vi "UI Config Controls.vi"(8 "Error In":errorcluster, 10 "UI Configuration":T1, 11 "UI Data":T2) -> (0 "Error Out":errorcluster, 3 "UI Data 2":T2)   [LabVIEW 2015]
uses:
  controls/UI Data.ctl
  controls/Instruments.ctl
  controls/UI Config.ctl
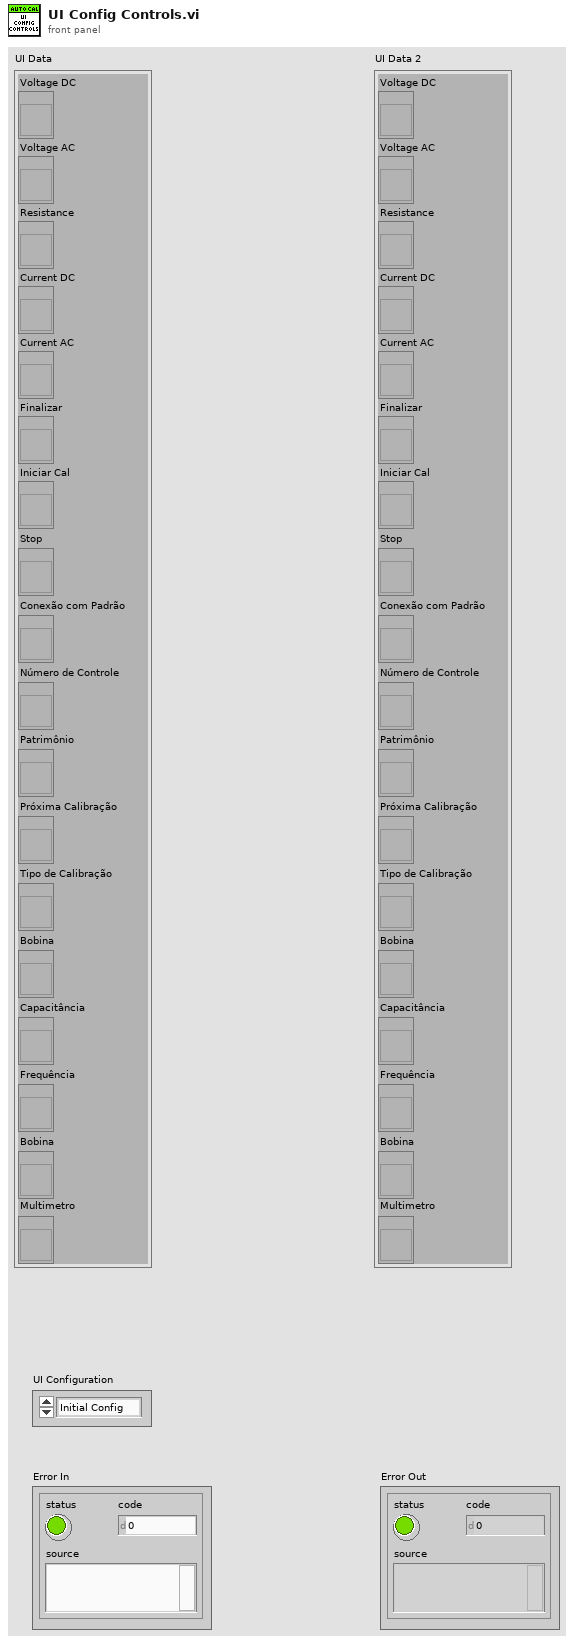
[diagram p1: front panel]
types:
  T1 = typedef "UI Config.ctl" = enum16{"Initial Config", "Calibration Config"}
  T2 = typedef "UI Data.ctl" = cluster{"Voltage DC":refnum<vi>, "Voltage AC":refnum<vi>, "Resistance":refnum<vi>, "Current DC":refnum<vi>, "Current AC":refnum<vi>, "Finalizar":refnum<vi>, "Iniciar Cal":refnum<vi>, "Stop":refnum<vi>, "Conexão com Padrão":refnum<vi>, "Número de Controle":refnum<vi>, "Patrimônio":refnum<vi>, "Próxima Calibração":refnum<vi>, "Tipo de Calibração":refnum<vi>, "Bobina":refnum<vi>, "Capacitância":refnum<vi>, "Frequência":refnum<vi>, "Bobina":refnum<vi>, "Multimetro":refnum<vi>}
  T3 = enum8{"Enabled", "Disabled", "Disabled and Grayed Out"}
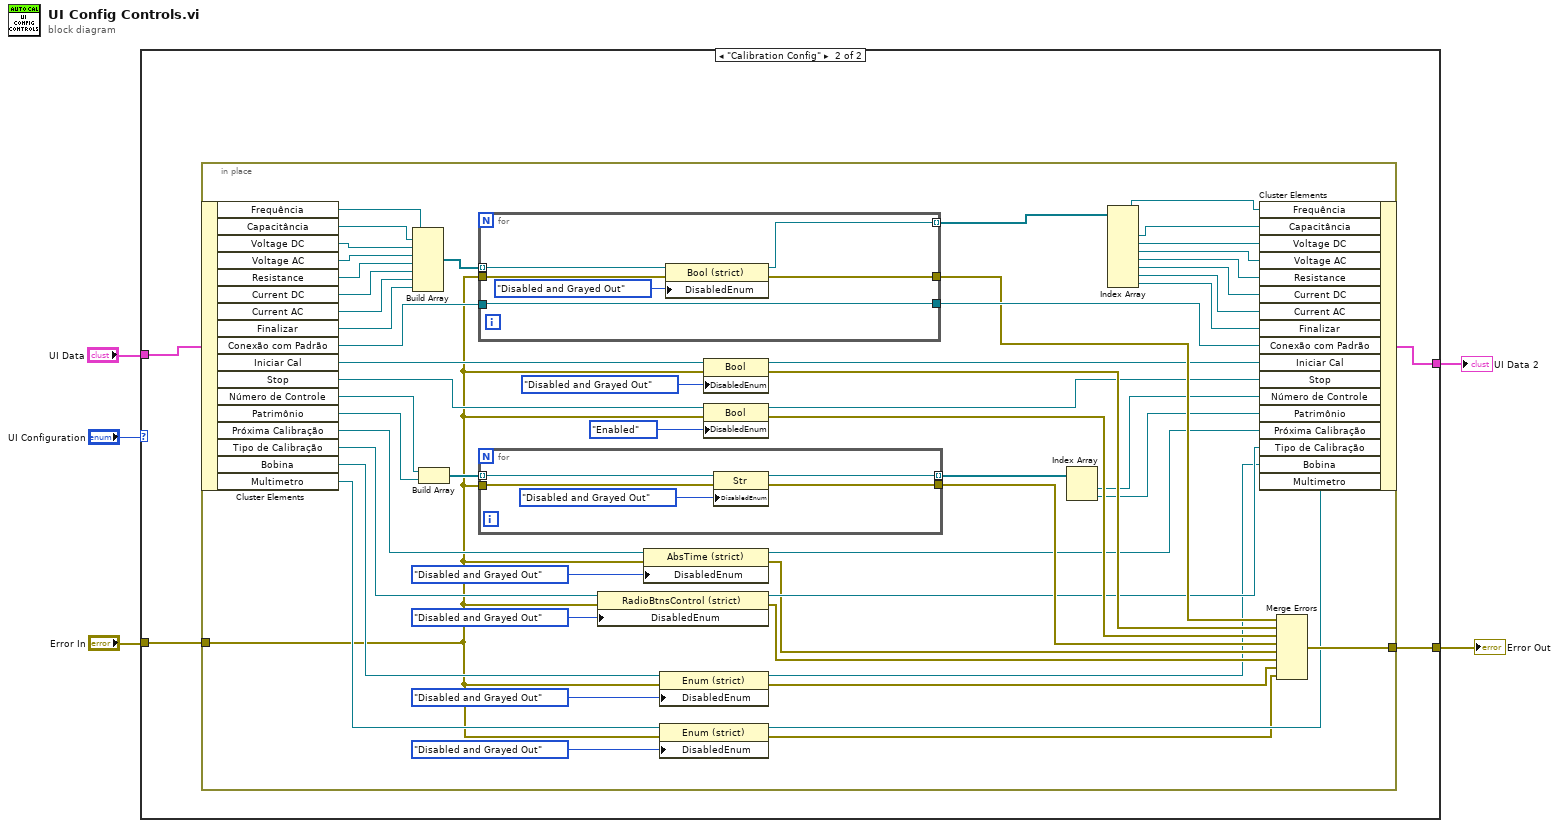
[diagram p0: block diagram]
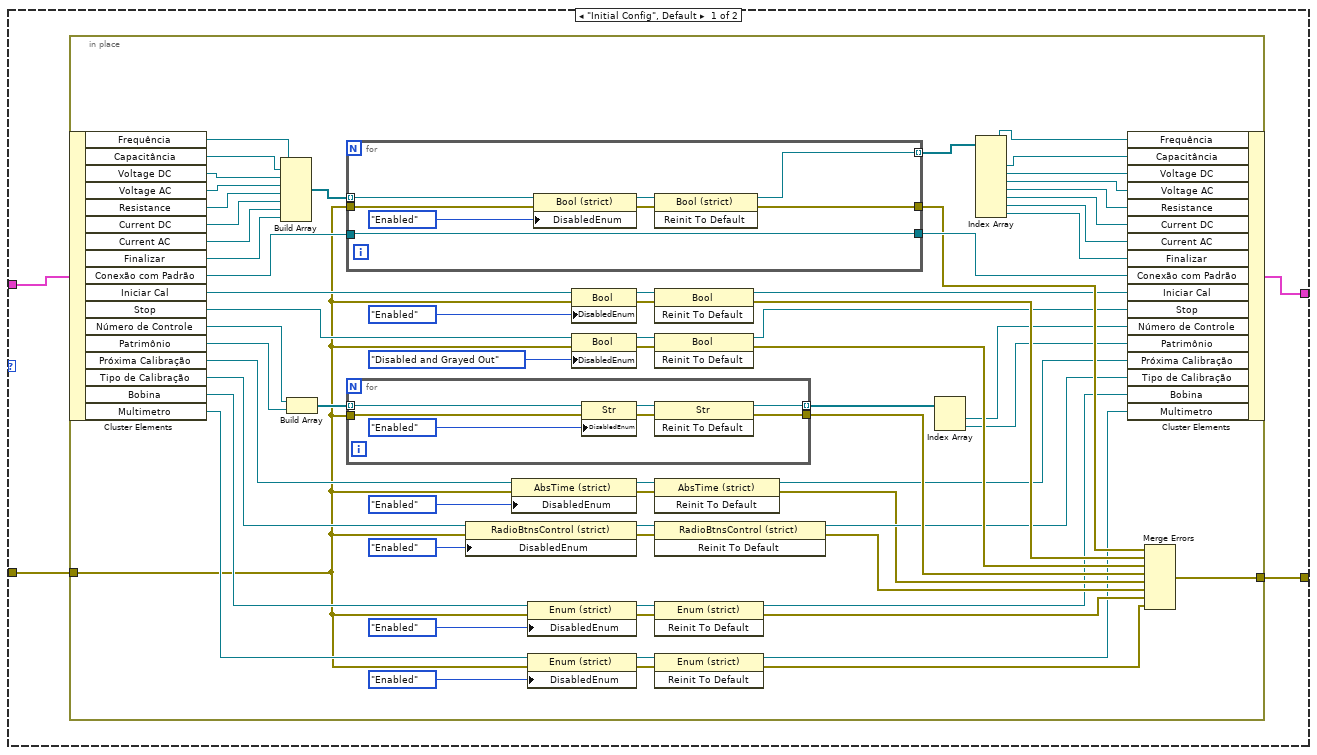
[diagram p2: hidden frame]
diagram:
  n1 = case shown="\"Calibration Config\"" "UI Configuration" {
    tunnel: "UI Data" -> [w9 w94]
    tunnel: [w8 w93] -> w4
    tunnel: "Error In" -> [w7 w92]
    tunnel: [w6 w91] -> w1
    frame "Initial Config", Default {
      n2 = in-place {
        in-place-border: w7 -> [w16]
        in-place-border: [w57] -> w6
        n3 = in-place-cluster #1(w9) -> ("Frequência"=w11:refnum<vi>, "Capacitância"=w13:refnum<vi>, "Voltage DC"=w75:refnum<vi>, "Voltage AC"=w74:refnum<vi>, "Resistance"=w73:refnum<vi>, "Current DC"=w72:refnum<vi>, "Current AC"=w71:refnum<vi>, "Finalizar"=w70:refnum<vi>, "Conexão com Padrão"=w61:refnum<vi>, "Iniciar Cal"=w51:refnum<vi>, "Stop"=w52:refnum<vi>, "Número de Controle"=w42:refnum<vi>, "Patrimônio"=w41:refnum<vi>, "Próxima Calibração"=w36:refnum<vi>, "Tipo de Calibração"=w32:refnum<vi>, "Bobina"=w23:refnum<vi>, "Multimetro"=w17:refnum<vi>)
        n4 = Build Array(w11, w13, w75, w74, w73, w72, w71, w70) -> (w69:refnum<vi>[])
        n5 = Build Array(w42, w41) -> (w40:refnum<vi>[])
        n6 = for {
          tunnel: w69 -> [w90] mode=indexing
          tunnel: w16 -> [w88]
          tunnel: [w85] -> w68 mode=indexing
          tunnel: w61 -> [w84]
          tunnel: [w84] -> w60
          tunnel: [w83] -> w59
          n7 = property class="Bool (strict)"(reference=w90, error in=w88, "DisabledEnum"=T3."Enabled" ("Disabled")) -> (reference out=w87:refnum<vi>, error out=w86:errorcluster)
          n8 = invoke class="Bool (strict)" method="Reinit To Default"(reference=w87, error in=w86) -> (reference out=w85:refnum<vi>, error out=w83:errorcluster)  [unwired: 1 in, 1 out]
        }
        n9 = for {
          tunnel: w40 -> [w82] mode=indexing
          tunnel: w16 -> [w80]
          tunnel: [w77] -> w39 mode=indexing
          tunnel: [w76] -> w31
          n10 = property class="Str"(reference=w82, error in=w80, "DisabledEnum"=T3."Enabled" ("Disabled")) -> (reference out=w79:refnum<vi>, error out=w78:errorcluster)
          n11 = invoke class="Str" method="Reinit To Default"(reference=w79, error in=w78) -> (reference out=w77:refnum<vi>, error out=w76:errorcluster)  [unwired: 1 in, 1 out]
        }
        n12 = property class="RadioBtnsControl (strict)"(reference=w32, error in=w16, "DisabledEnum"=T3."Enabled" ("Disabled")) -> (reference out=w33:refnum<vi>, error out=w35:errorcluster)
        n13 = property class="AbsTime (strict)"(reference=w36, error in=w16, "DisabledEnum"=T3."Enabled" ("Disabled")) -> (reference out=w45:refnum<vi>, error out=w43:errorcluster)
        n14 = property class="Enum (strict)"(reference=w23, error in=w16, "DisabledEnum"=T3."Enabled" ("Disabled")) -> (reference out=w25:refnum<vi>, error out=w24:errorcluster)
        n15 = property class="Enum (strict)"(reference=w17, error in=w16, "DisabledEnum"=T3."Enabled" ("Disabled")) -> (reference out=w19:refnum<vi>, error out=w20:errorcluster)
        n16 = property class="Bool"(reference=w51, error in=w16, "DisabledEnum"=T3."Enabled" ("Disabled")) -> (reference out=w46:refnum<vi>, error out=w56:errorcluster)
        n17 = property class="Bool"(reference=w52, error in=w16, "DisabledEnum"=T3."Disabled and Grayed Out" ("Disabled")) -> (reference out=w47:refnum<vi>, error out=w53:errorcluster)
        n18 = invoke class="Bool" method="Reinit To Default"(reference=w46, error in=w56) -> (reference out=w50:refnum<vi>, error out=w58:errorcluster)  [unwired: 1 in, 1 out]
        n19 = invoke class="Bool" method="Reinit To Default"(reference=w47, error in=w53) -> (reference out=w49:refnum<vi>, error out=w48:errorcluster)  [unwired: 1 in, 1 out]
        n20 = invoke class="AbsTime (strict)" method="Reinit To Default"(reference=w45, error in=w43) -> (reference out=w30:refnum<vi>, error out=w28:errorcluster)  [unwired: 1 in, 1 out]
        n21 = invoke class="RadioBtnsControl (strict)" method="Reinit To Default"(reference=w33, error in=w35) -> (reference out=w29:refnum<vi>, error out=w27:errorcluster)  [unwired: 1 in, 1 out]
        n22 = invoke class="Enum (strict)" method="Reinit To Default"(reference=w25, error in=w24) -> (reference out=w22:refnum<vi>, error out=w21:errorcluster)  [unwired: 1 in, 1 out]
        n23 = invoke class="Enum (strict)" method="Reinit To Default"(reference=w19, error in=w20) -> (reference out=w15:refnum<vi>, error out=w14:errorcluster)  [unwired: 1 in, 1 out]
        n24 = Index Array(array=w39) -> (element #1=w38:refnum<vi>, element #2=w37:refnum<vi>)  [unwired: 2 in]
        n25 = Index Array(array=w68) -> (element #1=w10:refnum<vi>, element #2=w12:refnum<vi>, element #3=w67:refnum<vi>, element #4=w66:refnum<vi>, element #5=w65:refnum<vi>, element #6=w64:refnum<vi>, element #7=w63:refnum<vi>, element #8=w62:refnum<vi>)  [unwired: 8 in]
        n26 = in-place-cluster #1("Frequência"=w10, "Capacitância"=w12, "Voltage DC"=w67, "Voltage AC"=w66, "Resistance"=w65, "Current DC"=w64, "Current AC"=w63, "Finalizar"=w62, "Conexão com Padrão"=w60, "Iniciar Cal"=w50, "Stop"=w49, "Número de Controle"=w38, "Patrimônio"=w37, "Próxima Calibração"=w30, "Tipo de Calibração"=w29, "Bobina"=w22, "Multimetro"=w15) -> (w8:T2)
        n27 = Merge Errors(w59, w58, w48, w31, w28, w27, w21, w14) -> (w57:errorcluster)
      }
    }
    frame "Calibration Config" {
      n28 = in-place {
        in-place-border: w92 -> [w101]
        in-place-border: [w130] -> w91
        n29 = in-place-cluster #2(w94) -> ("Frequência"=w96:refnum<vi>, "Capacitância"=w98:refnum<vi>, "Voltage DC"=w148:refnum<vi>, "Voltage AC"=w147:refnum<vi>, "Resistance"=w146:refnum<vi>, "Current DC"=w145:refnum<vi>, "Current AC"=w144:refnum<vi>, "Finalizar"=w143:refnum<vi>, "Conexão com Padrão"=w134:refnum<vi>, "Iniciar Cal"=w126:refnum<vi>, "Stop"=w127:refnum<vi>, "Número de Controle"=w121:refnum<vi>, "Patrimônio"=w120:refnum<vi>, "Próxima Calibração"=w115:refnum<vi>, "Tipo de Calibração"=w113:refnum<vi>, "Bobina"=w106:refnum<vi>, "Multimetro"=w102:refnum<vi>)
        n30 = Build Array(w96, w98, w148, w147, w146, w145, w144, w143) -> (w142:refnum<vi>[])
        n31 = Build Array(w121, w120) -> (w119:refnum<vi>[])
        n32 = for {
          tunnel: w142 -> [w159] mode=indexing
          tunnel: w101 -> [w157]
          tunnel: [w156] -> w141 mode=indexing
          tunnel: w134 -> [w155]
          tunnel: [w155] -> w133
          tunnel: [w154] -> w132
          n33 = property class="Bool (strict)"(reference=w159, error in=w157, "DisabledEnum"=T3."Disabled and Grayed Out" ("Disabled")) -> (reference out=w156:refnum<vi>, error out=w154:errorcluster)
        }
        n34 = for {
          tunnel: w119 -> [w153] mode=indexing
          tunnel: w101 -> [w151]
          tunnel: [w150] -> w118 mode=indexing
          tunnel: [w149] -> w112
          n35 = property class="Str"(reference=w153, error in=w151, "DisabledEnum"=T3."Disabled and Grayed Out" ("Disabled")) -> (reference out=w150:refnum<vi>, error out=w149:errorcluster)
        }
        n36 = property class="RadioBtnsControl (strict)"(reference=w113, error in=w101, "DisabledEnum"=T3."Disabled and Grayed Out" ("Disabled")) -> (reference out=w110:refnum<vi>, error out=w108:errorcluster)
        n37 = property class="AbsTime (strict)"(reference=w115, error in=w101, "DisabledEnum"=T3."Disabled and Grayed Out" ("Disabled")) -> (reference out=w111:refnum<vi>, error out=w109:errorcluster)
        n38 = property class="Enum (strict)"(reference=w106, error in=w101, "DisabledEnum"=T3."Disabled and Grayed Out" ("Disabled")) -> (reference out=w105:refnum<vi>, error out=w104:errorcluster)
        n39 = property class="Enum (strict)"(reference=w102, error in=w101, "DisabledEnum"=T3."Disabled and Grayed Out" ("Disabled")) -> (reference out=w100:refnum<vi>, error out=w99:errorcluster)
        n40 = property class="Bool"(reference=w126, error in=w101, "DisabledEnum"=T3."Disabled and Grayed Out" ("Disabled")) -> (reference out=w125:refnum<vi>, error out=w131:errorcluster)
        n41 = property class="Bool"(reference=w127, error in=w101, "DisabledEnum"=T3."Enabled" ("Disabled")) -> (reference out=w124:refnum<vi>, error out=w123:errorcluster)
        n42 = Index Array(array=w118) -> (element #1=w117:refnum<vi>, element #2=w116:refnum<vi>)  [unwired: 2 in]
        n43 = Index Array(array=w141) -> (element #1=w95:refnum<vi>, element #2=w97:refnum<vi>, element #3=w140:refnum<vi>, element #4=w139:refnum<vi>, element #5=w138:refnum<vi>, element #6=w137:refnum<vi>, element #7=w136:refnum<vi>, element #8=w135:refnum<vi>)  [unwired: 8 in]
        n44 = in-place-cluster #2("Frequência"=w95, "Capacitância"=w97, "Voltage DC"=w140, "Voltage AC"=w139, "Resistance"=w138, "Current DC"=w137, "Current AC"=w136, "Finalizar"=w135, "Conexão com Padrão"=w133, "Iniciar Cal"=w125, "Stop"=w124, "Número de Controle"=w117, "Patrimônio"=w116, "Próxima Calibração"=w111, "Tipo de Calibração"=w110, "Bobina"=w105, "Multimetro"=w100) -> (w93:T2)
        n45 = Merge Errors(w132, w131, w123, w112, w109, w108, w104, w99) -> (w130:errorcluster)
      }
    }
  }
  "UI Data 2" <- w4
  "Error Out" <- w1
